vi "Read Number of children.vi"(8 "error in (no error)":errorcluster, 11 "Test Actor in":refnum<class "Example Actor.lvclass">) -> (0 "error out":errorcluster, 2 "Number of children":i32, 3 "Test Actor out":refnum<class "Example Actor.lvclass">)   [LabVIEW 2020, in "Example Actor.lvlib" / "Example Actor.lvclass"]
uses:
  Example Actor.lvclass
  Example Actor.lvclass/Example Actor.ctl
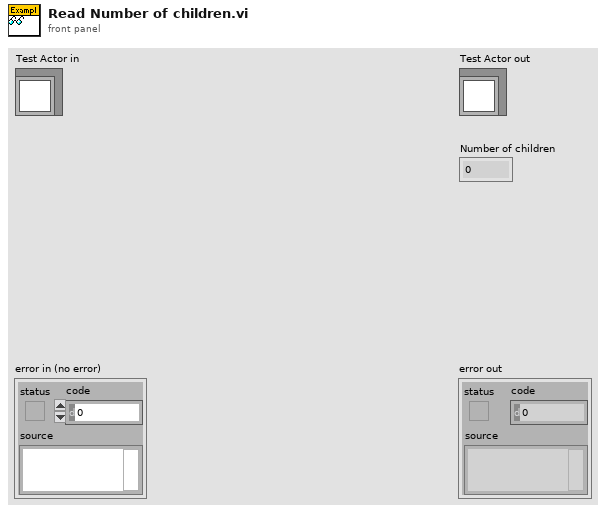
[diagram p1: front panel]
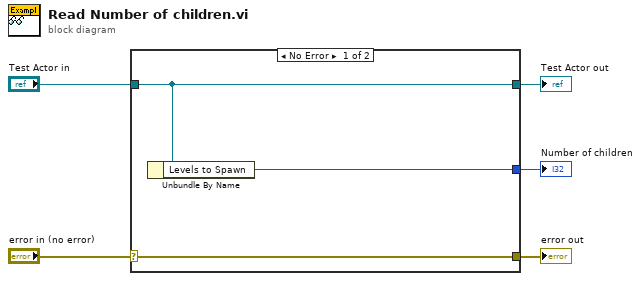
[diagram p0: block diagram]
diagram:
  n1 = case shown="No Error" "error in (no error)" {
    selector: "error in (no error)" -> [w8 w9]
    tunnel: [w8 w9] -> w4
    tunnel: [w7 w10] -> w2
    tunnel: "Test Actor in" -> [w7 w10]
    tunnel: [w6 _] -> w1
    frame No Error {
      n2 = Unbundle By Name(w7) -> ("Levels to Spawn"=w6:i32)
    }
    frame Error {
    }
  }
  "error out" <- w4
  "Test Actor out" <- w2
  "Number of children" <- w1
